vi "BuildWindow.vi"(7 "Init (f)":bool, 8 "error in (no error)":errorcluster, 10 "clSampleData":T1 {"Timestamp" format="%.6f"}, 11 "AnalysisPluginsBase in":refnum<class "AnalysisPluginsBase.lvclass">) -> (0 "error out":errorcluster, 3 "AnalysisPluginsBase out":refnum<class "AnalysisPluginsBase.lvclass">)   [LabVIEW 2014]
uses:
  AnalysisPluginsBase.lvclass
  Typedefs/clSampleData.ctl
panel:
  out "WindowValid":bool
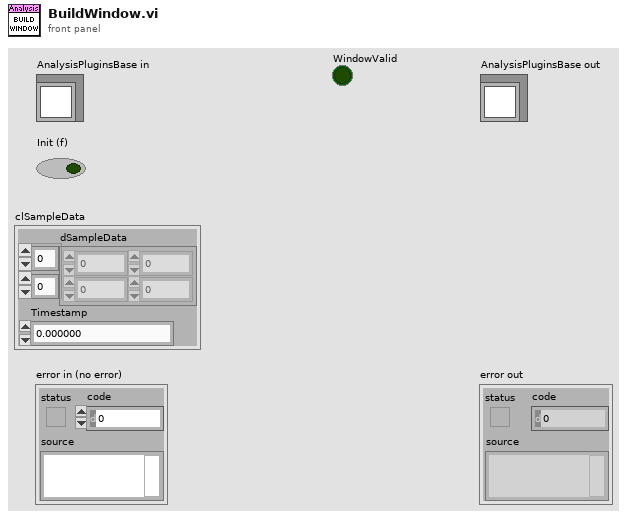
[diagram p1: front panel]
types:
  T1 = typedef "AnalysisPlugins.lvlib/AnalysisPluginsBase.lvclass/clSampleData.ctl" = cluster{"dSampleData":dbl[][], "Timestamp":ext}
  T2 = typedef "AnalysisPlugins.lvlib/AnalysisPluginsBase.lvclass/clConfig.ctl" = cluster{"F0":u32, "SettlingTime":dbl, "AnalysisCycles":dbl, "SampleRate":dbl, "NumChannels":u32}
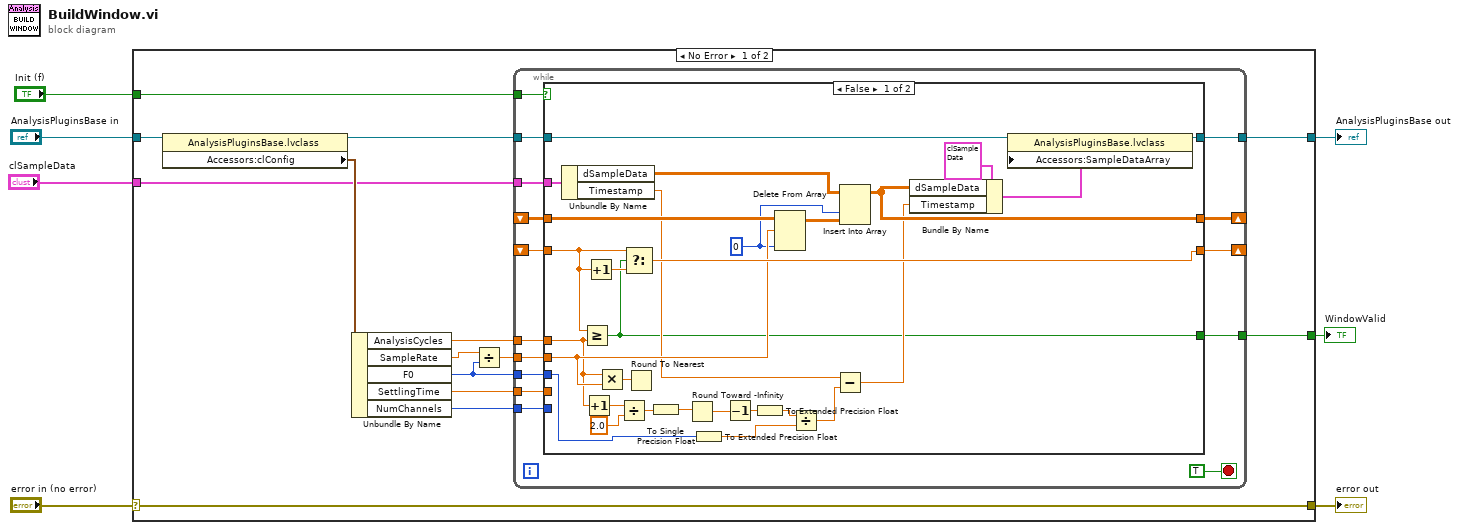
[diagram p0: block diagram]
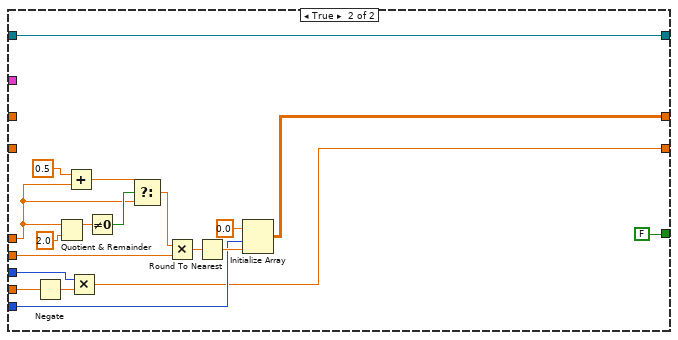
[diagram p2: hidden frame]
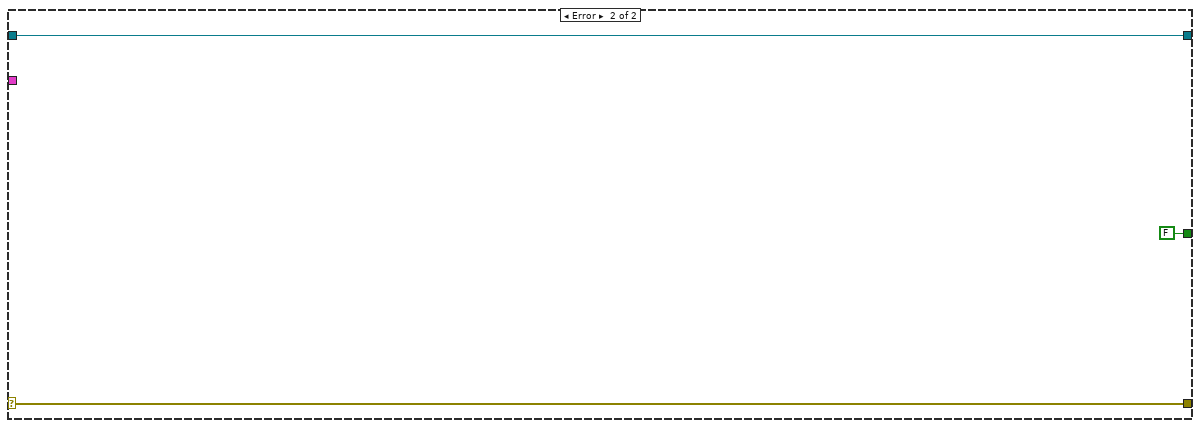
[diagram p3: hidden frame]
diagram:
  n1 = case shown="No Error" "error in (no error)" {
    selector: "error in (no error)" -> [w20 w87]
    tunnel: [w20 w87] -> w6
    tunnel: [w9 w86] -> w4
    tunnel: "AnalysisPluginsBase in" -> [w21 w86]
    tunnel: "Init (f)" -> [w16 _]
    tunnel: "clSampleData" -> [w10 _]
    tunnel: [w8 FALSE] -> w1
    frame No Error {
      n2 = property class="AnalysisPluginsBase.lvclass"(reference=w21) -> (reference out=w11:refnum<class "AnalysisPluginsBase.lvclass">, "Accessors:clConfig"=w19:T2)  [unwired: 1 in, 1 out]
      n3 = Unbundle By Name(w19) -> ("AnalysisCycles"=w18:dbl, "SampleRate"=w15:dbl, "F0"=w14:u32, "SettlingTime"=w17:dbl, "NumChannels"=w12:u32)
      n4 = Divide(x=w15, y=w14) -> (x/y=w13:dbl)
      n5 = while {
        tunnel: w18 -> [w34]
        tunnel: w13 -> [w33]
        tunnel: w14 -> [w32]
        tunnel: w17 -> [w31]
        tunnel: w16 -> [w35]
        tunnel: w12 -> [w30]
        shift-right: [w29] -> _
        shift-left: _ -> [w24]
        shift-right: [w28] -> _
        shift-left: _ -> [w25]
        tunnel: w11 -> [w27]
        tunnel: w10 -> [w26]
        tunnel: [w23] -> w9
        tunnel: [w22] -> w8
        stop <- TRUE stop-if-true
        n6 = case shown="False" w35 {
          tunnel: w34 -> [w55 w79]
          tunnel: w33 -> [w59 w78]
          tunnel: w32 -> [w47 w70]
          tunnel: w31 -> [_ w72]
          tunnel: w30 -> [_ w74]
          tunnel: [w61 w69] -> w29
          tunnel: [w43 w68] -> w28
          tunnel: w27 -> [w45 w67]
          tunnel: w26 -> [w65 _]
          tunnel: w25 -> [w64 _]
          tunnel: w24 -> [w62 _]
          tunnel: [w41 w67] -> w23
          tunnel: [w37 FALSE] -> w22
          frame False {
            w56 = 0 ("disabled index (col)")
            n7 = Unbundle By Name(w65) -> ("dSampleData"=w57:dbl[][], "Timestamp"=w39:ext)
            n8 = Greater Or Equal?(x=w62, y=w55) -> (x >= y?=w37:bool)
            n9 = Increment(x=w55) -> (x+1=w54:dbl)
            n10 = Increment(x=w62) -> (x+1=w63:dbl)
            n11 = Multiply(x=w55, y=w59) -> (x*y=w60:dbl)
            n12 = Divide(x=w54, y=2.0) -> (x/y=w52:dbl)
            n13 = Select(t=w62, s=w37, f=w63) -> (s? t:f=w61:dbl)
            n14 = Round To Nearest(number=w60) -> ()  [unwired: 1 out]
            n15 = To Single Precision Float(number=w52) -> (single precision float=w51:sgl)
            n16 = Round Toward -Infinity(1:w51) -> (0:w50:sgl)
            n17 = To Extended Precision Float(1:w47) -> (0:w46:ext)
            n18 = Decrement(x=w50) -> (x-1=w49:sgl)
            n19 = To Extended Precision Float(1:w49) -> (0:w48:ext)
            n20 = Delete From Array(array=w64, length=w59, index (col)=w56) -> (array with subset deleted=w58:dbl[][])  [unwired: 1 in, 1 out]
            n21 = Divide(x=w48, y=w46) -> (x/y=w40:ext)
            n22 = Subtract(x=w39, y=w40) -> (x-y=w38:ext)
            n23 = Insert Into Array(array=w57, index (col)=w56, new element=w58) -> (w43:dbl[][])  [unwired: 1 in]
            n24 = Bundle By Name(cluster=T1 {"dSampleData"=[], "Timestamp"=0.0} ("clSampleData"), "dSampleData"=w43, "Timestamp"=w38) -> (w42:T1)
            n25 = property class="AnalysisPluginsBase.lvclass"(reference=w45, "Accessors:SampleDataArray"=w42) -> (reference out=w41:refnum<class "AnalysisPluginsBase.lvclass">)  [unwired: 1 in, 1 out]
          }
          frame True {
            n26 = Negate(x=w72) -> (-x=w71:dbl)
            n27 = Quotient & Remainder(x=w79, y=2.0) -> (x-y*floor(x/y)=w84:dbl)  [unwired: 1 out]
            n28 = Add(x=0.5, y=w79) -> (x+y=w82:dbl)
            n29 = Multiply(x=w70, y=w71) -> (x*y=w69:dbl)
            n30 = Not Equal To 0?(x=w84) -> (x != 0?=w80:bool)
            n31 = Select(t=w82, s=w80, f=w79) -> (s? t:f=w77:dbl)
            n32 = Multiply(x=w77, y=w78) -> (x*y=w76:dbl)
            n33 = Round To Nearest(number=w76) -> (nearest integer value=w75:dbl)
            n34 = Initialize Array(0.0 ("element"), w74, w75) -> (w68:dbl[][])
          }
        }
      }
    }
    frame Error {
    }
  }
  "error out" <- w6
  "AnalysisPluginsBase out" <- w4
  "WindowValid" <- w1
